vi "Create Lib in Project.vi"(8 "error in (no error)":errorcluster, 9 "Save Path":path, 10 "Library Name":string, 11 "Project in":refnum<vi>) -> (0 "error out":errorcluster, 2 "Library out":refnum<vi>, 3 "Project out":refnum<vi>)   [LabVIEW 2019, in "gRPC Scripting Tools.lvlib"]
uses:
  gRPC Scripting Tools.lvlib
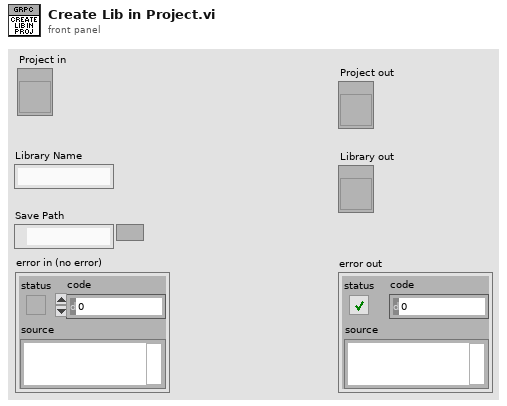
[diagram p1: front panel]
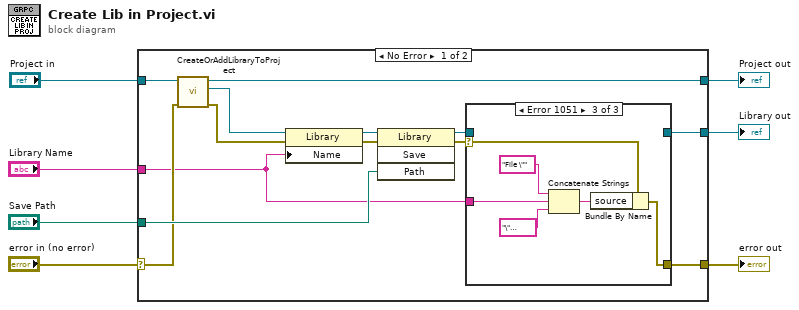
[diagram p0: block diagram]
diagram:
  n1 = case shown="No Error" "error in (no error)" {
    selector: "error in (no error)" -> [w14 w31]
    tunnel: "Save Path" -> [w20 _]
    tunnel: "Library Name" -> [w9 _]
    tunnel: "Project in" -> [w17 w30]
    tunnel: [w11 _] -> w5
    tunnel: [w10 w31] -> w4
    tunnel: [w8 w30] -> w1
    frame No Error {
      n2 = call <vilib>:"CreateOrAddLibraryToProject.vi"("error in (no error)"=w14, "Project Reference In (Create New)"=w17) -> ("error out"=w18:errorcluster, "Library Reference Out"=w15:refnum<vi>, "Project Reference Out"=w8:refnum<vi>)  [unwired: 7 in]
      n3 = property class="Library"(reference=w15, error in=w18, "Name"=w9) -> (reference out=w16:refnum<vi>, error out=w19:errorcluster)
      n4 = invoke class="Library" method="Save"(reference=w16, error in=w19, "Path"=w20) -> (reference out=w12:refnum<vi>, error out=w13:errorcluster)  [unwired: 1 in, 2 out]
      n5 = case shown="Error 1051" w13 {
        selector: w13 -> [w21 w23 w29]
        tunnel: w12 -> [w22 _ _]
        tunnel: [w22 _ _] -> w11
        tunnel: [w21 w23 w28] -> w10
        tunnel: w9 -> [_ _ w26]
        frame No Error {
        }
        frame Default {
        }
        frame Error {
          n6 = Concatenate Strings("File \"" ("source"), w26, "\" already exists in the project." ("string")) -> (w24:string)
          n7 = Bundle By Name(cluster=w29, "source"=w24) -> (w28:errorcluster)
        }
      }
    }
    frame Error {
    }
  }
  "Library out" <- w5
  "error out" <- w4
  "Project out" <- w1
